vi "RichToFlatnixnet_grpc_WriteFrameRequest.vi"(5 "OutputClusterType":T1, 11 "InputCluster":T11) -> (3 "OutputCluster":T1)   [LabVIEW 2025, in "grpc-xnet_client.lvlib"]
uses:
  grpc-xnet_client.lvlib
  nixnet_grpc_WriteFrameRequest.ctl
  nixnet_grpc_WriteFrameRequest_timeout_enum/nixnet_grpc_WriteFrameRequest_timeout_enum.lvclass
  nidevice_grpc_Session.ctl
  nixnet_grpc_FrameBufferRequest.ctl
  nixnet_grpc_FrameBufferRequest_frame/nixnet_grpc_FrameBufferRequest_frame.lvclass
  nixnet_grpc_WriteFrameRequest_Flat.ctl
  nidevice_grpc_Session_Flat.ctl
  nixnet_grpc_FrameBufferRequest_Flat.ctl
  nixnet_grpc_FrameRequest_Flat.ctl
  nixnet_grpc_FrameType.ctl
  nixnet_grpc_FrameFlags.ctl
  nixnet_grpc_EnetFrameRequest_Flat.ctl
  nixnet_grpc_EnetFrameType.ctl
  nixnet_grpc_EnetFlags.ctl
  nixnet_grpc_TimeOut.ctl
  nixnet_grpc_WriteFrameRequest_timeout_enum/nixnet_grpc_WriteFrameRequest_timeout_enum.lvclass/nixnet_grpc_WriteFrameRequest_timeout_enum.ctl
  nixnet_grpc_FrameBufferRequest_frame/nixnet_grpc_FrameBufferRequest_frame.lvclass/nixnet_grpc_FrameBufferRequest_frame.ctl
  nixnet_grpc_EnetFrameRequest_type_enum/nixnet_grpc_EnetFrameRequest_type_enum.lvclass/nixnet_grpc_EnetFrameRequest_type_enum.ctl
  nixnet_grpc_FrameRequest_type_enum/nixnet_grpc_FrameRequest_type_enum.lvclass/nixnet_grpc_FrameRequest_type_enum.ctl
  nixnet_grpc_FrameBufferRequest_frame/Getcan.vi
  RichToFlatnixnet_grpc_FrameRequest.vi
  nixnet_grpc_FrameBufferRequest_frame/Getlin.vi
  nixnet_grpc_FrameBufferRequest_frame/Getflex_ray.vi
  nixnet_grpc_FrameBufferRequest_frame/Getj1939.vi
  nixnet_grpc_FrameBufferRequest_frame/Getenet.vi
  RichToFlatnixnet_grpc_EnetFrameRequest.vi
  nixnet_grpc_FrameRequest_type_enum/Gettype.vi
  nixnet_grpc_FrameRequest_type_enum/Gettype_raw.vi
  nixnet_grpc_EnetFrameRequest_type_enum/Gettype.vi
  nixnet_grpc_EnetFrameRequest_type_enum/Gettype_raw.vi
  nixnet_grpc_EnetFrameRequest_type_enum/nixnet_grpc_EnetFrameRequest_type_enum.lvclass
  nixnet_grpc_FrameRequest_type_enum/nixnet_grpc_FrameRequest_type_enum.lvclass
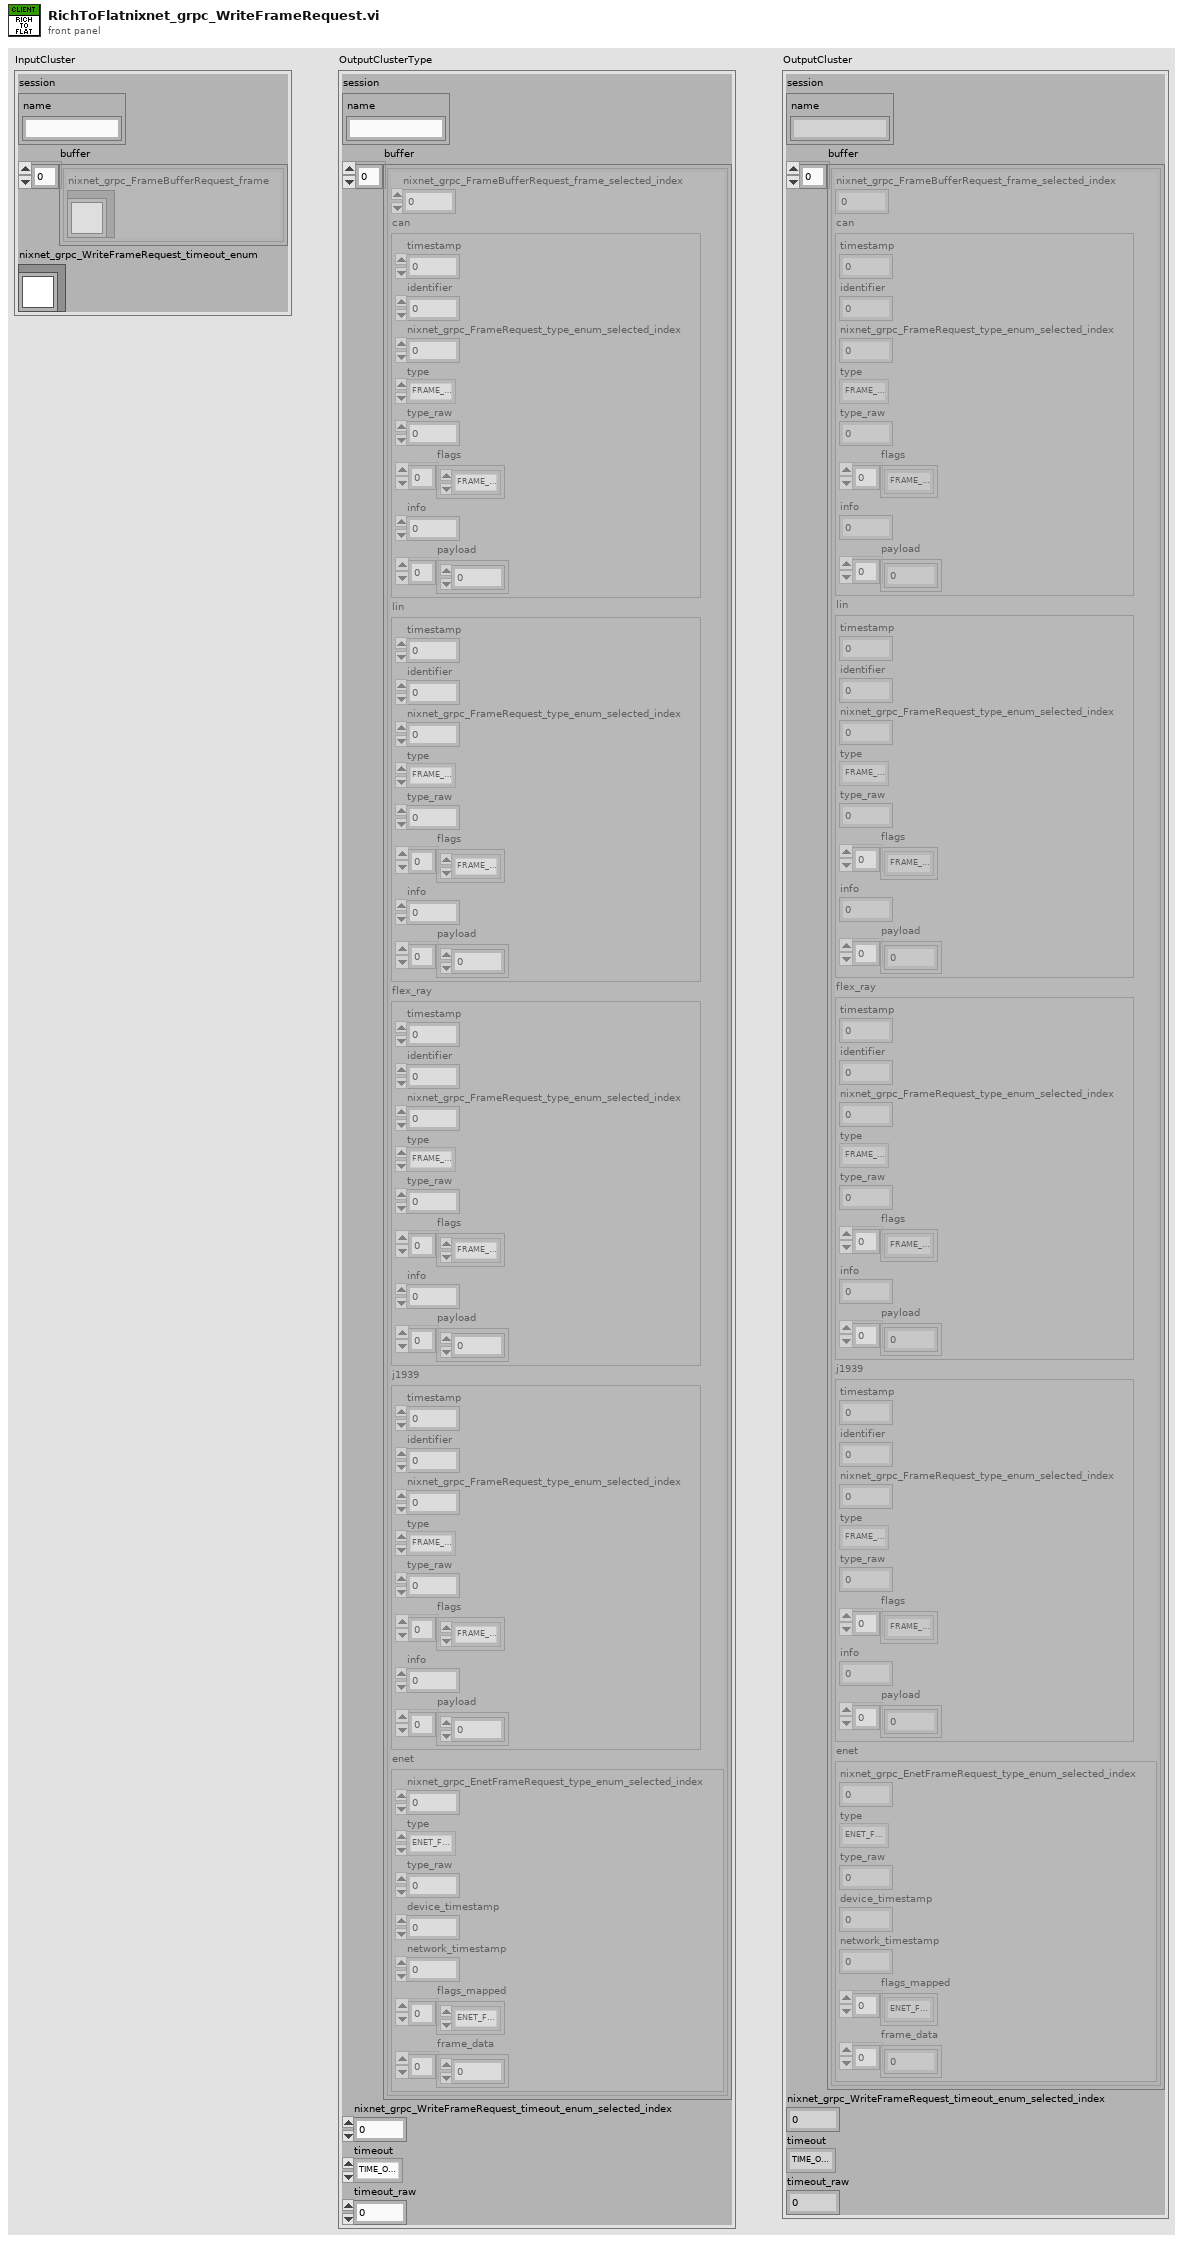
[diagram p1: front panel]
types:
  T1 = typedef "grpc-xnet_client.lvlib/nixnet_grpc_WriteFrameRequest_Flat.ctl" = cluster{"session":T2, "buffer":T3[], "nixnet_grpc_WriteFrameRequest_timeout_enum_selected_index":i32, "timeout":T10, "timeout_raw":dbl}
  T2 = typedef "grpc-xnet_client.lvlib/nidevice_grpc_Session_Flat.ctl" = cluster{"name":string}
  T3 = typedef "grpc-xnet_client.lvlib/nixnet_grpc_FrameBufferRequest_Flat.ctl" = cluster{"nixnet_grpc_FrameBufferRequest_frame_selected_index":i32, "can":T4, "lin":T4, "flex_ray":T4, "j1939":T4, "enet":T7}
  T4 = typedef "grpc-xnet_client.lvlib/nixnet_grpc_FrameRequest_Flat.ctl" = cluster{"timestamp":u64, "identifier":u32, "nixnet_grpc_FrameRequest_type_enum_selected_index":i32, "type":T5, "type_raw":u32, "flags":T6[], "info":u32, "payload":u8[]}
  T5 = typedef "grpc-xnet_client.lvlib/nixnet_grpc_FrameType.ctl" = enum32{"FRAME_TYPE_CAN_DATA", "FRAME_TYPE_CAN_REMOTE", "FRAME_TYPE_CAN_BUS_ERROR", "FRAME_TYPE_CAN20_DATA", "FRAME_TYPE_CANFD_DATA", "FRAME_TYPE_CANFDBRS_DATA", "FRAME_TYPE_FLEX_RAY_DATA", "FRAME_TYPE_FLEX_RAY_NULL", "FRAME_TYPE_FLEX_RAY_SYMBOL", "FRAME_TYPE_LIN_DATA", "FRAME_TYPE_LIN_BUS_ERROR", "FRAME_TYPE_LIN_NO_RESPONSE", "FRAME_TYPE_J1939_DATA", "FRAME_TYPE_SPECIAL_DELAY", "FRAME_TYPE_SPECIAL_LOG_TRIGGER", "FRAME_TYPE_SPECIAL_START_TRIGGER"}
  T6 = typedef "grpc-xnet_client.lvlib/nixnet_grpc_FrameFlags.ctl" = enum32{"FRAME_FLAGS_UNSPECIFIED", "FRAME_FLAGS_FLEX_RAY_STARTUP", "FRAME_FLAGS_FLEX_RAY_SYNC", "FRAME_FLAGS_FLEX_RAY_PREAMBLE", "FRAME_FLAGS_FLEX_RAY_CH_A", "FRAME_FLAGS_FLEX_RAY_CH_B", "FRAME_FLAGS_LIN_EVENT_SLOT", "FRAME_FLAGS_TRANSMIT_ECHO"}
  T7 = typedef "grpc-xnet_client.lvlib/nixnet_grpc_EnetFrameRequest_Flat.ctl" = cluster{"nixnet_grpc_EnetFrameRequest_type_enum_selected_index":i32, "type":T8, "type_raw":u32, "device_timestamp":u64, "network_timestamp":u64, "flags_mapped":T9[], "frame_data":u8[]}
  T8 = typedef "grpc-xnet_client.lvlib/nixnet_grpc_EnetFrameType.ctl" = enum32{"ENET_FRAME_TYPE_DATA", "ENET_FRAME_TYPE_DELAY", "ENET_FRAME_TYPE_FUTURE_TIME_WAIT"}
  T9 = typedef "grpc-xnet_client.lvlib/nixnet_grpc_EnetFlags.ctl" = enum32{"ENET_FLAGS_UNSPECIFIED", "ENET_FLAGS_TRANSMIT", "ENET_FLAGS_RECEIVE", "ENET_FLAGS_NETWORK_SYNCED", "ENET_FLAGS_ERROR"}
  T10 = typedef "grpc-xnet_client.lvlib/nixnet_grpc_TimeOut.ctl" = enum32{"TIME_OUT_NONE", "TIME_OUT_INFINITE"}
  T11 = typedef "grpc-xnet_client.lvlib/nixnet_grpc_WriteFrameRequest.ctl" = cluster{"session":T12, "buffer":T13[], "nixnet_grpc_WriteFrameRequest_timeout_enum":refnum<class "nixnet_grpc_WriteFrameRequest_timeout_enum.lvclass">}
  T12 = typedef "grpc-xnet_client.lvlib/nidevice_grpc_Session.ctl" = cluster{"name":string}
  T13 = typedef "grpc-xnet_client.lvlib/nixnet_grpc_FrameBufferRequest.ctl" = cluster{"nixnet_grpc_FrameBufferRequest_frame":refnum<class "nixnet_grpc_FrameBufferRequest_frame.lvclass">}
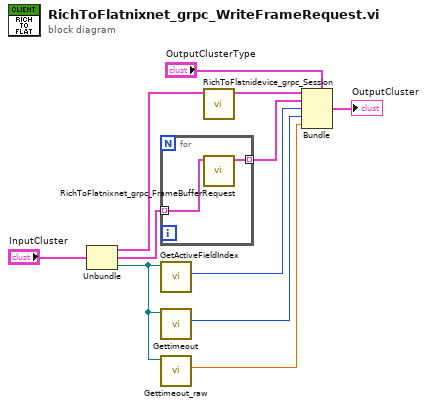
[diagram p0: block diagram]
diagram:
  n1 = Unbundle "Unbundle"("InputCluster") -> ("session"=w8:T12, "buffer"=w6:T13[], "nixnet_grpc_WriteFrameRequest_timeout_enum"=w4:refnum<class "nixnet_grpc_WriteFrameRequest_timeout_enum.lvclass">)
  n2 = for {
    tunnel: w6 -> [w13] mode=indexing
    tunnel: [w12] -> w5 mode=indexing
    n3 = call "RichToFlatnixnet_grpc_FrameBufferRequest.vi"("InputCluster"=w13) -> ("OutputCluster"=w12:T3)  [unwired: 10 in]
  }
  n4 = call "GetActiveFieldIndex.vi"("OneOfTemplate in"=w4) -> ("Active Field Index"=w3:i32)  [unwired: 8 in, 2 out]
  n5 = call "Gettimeout.vi"("OneOfTemplate in"=w4) -> ("Get_Val"=w2:T10)  [unwired: 8 in, 2 out]
  n6 = call "Gettimeout_raw.vi"("OneOfTemplate in"=w4) -> ("Get_Val"=w1:dbl)  [unwired: 8 in, 2 out]
  n7 = call "RichToFlatnidevice_grpc_Session.vi"("InputCluster"=w8) -> ("OutputCluster"=w7:T2)  [unwired: 10 in]
  n8 = Bundle "Bundle"(cluster="OutputClusterType", "session"=w7, "buffer"=w5, "nixnet_grpc_WriteFrameRequest_timeout_enum_selected_index"=w3, "timeout"=w2, "timeout_raw"=w1) -> (→"OutputCluster":T1)
